vi "test - NESTED Multiple nested read and write operations of submodules.vi"(8 "error in (no error)":errorcluster, 11 "TestCase in":refnum<class "csm-ini-variable-addon.lvclass">) -> (0 "error out":errorcluster, 3 "TestCase out":refnum<class "csm-ini-variable-addon.lvclass">)   [LabVIEW 2017, in "csm-ini-variable-addon.lvclass"]
uses:
  csm-ini-variable-addon.lvclass
  fd1f1403-f650-4147-a5d0-7fa8994ff20a.vi
  a890fef7-7f1d-42c9-b9db-12bb2b441289.vi
  25df91f5-a8e9-4b30-a15a-ad417606420d.vi
  4506128f-911b-4b09-9ad5-a28d51cf287f.vi
  fd1f1403-f650-4147-a5d0-7fa8994ff20a.vi/caddadbc-c5ad-445f-bfd7-34f99667ea02.vi
  <vilib>/Utility/error.llb/Clear Errors.vi
  a890fef7-7f1d-42c9-b9db-12bb2b441289.vi/5b17a956-d3a2-4fc5-bd5f-1f511fac3c4f.vi
  25df91f5-a8e9-4b30-a15a-ad417606420d.vi/a3ec2e19-b962-4b46-9572-7cb078ba8762.vi
  4506128f-911b-4b09-9ad5-a28d51cf287f.vi/14c6159a-6b3d-4974-8c79-afba77de3931.vi
  <vilib>/Utility/Data Type/Get Type Information.vi
  <userlib>/_NEVSTOP/Communicable State Machine(CSM)/addons/API-String-Arugments-Support/_Support/Data To SingleElementsArray_csm.vi
  <userlib>/_NEVSTOP/Communicable State Machine(CSM)/addons/API-String-Arugments-Support/_Support/Data To API String Arguments.vi
  INI-Static-Variable-Support/_Support/Parse Used Session and Name.vi
  INI-Static-Variable-Support/_Support/INI-FGV.vi
  INI-Static-Variable-Support/INI-Static-Variable-Support.lvlib
panel:
  out "text":string
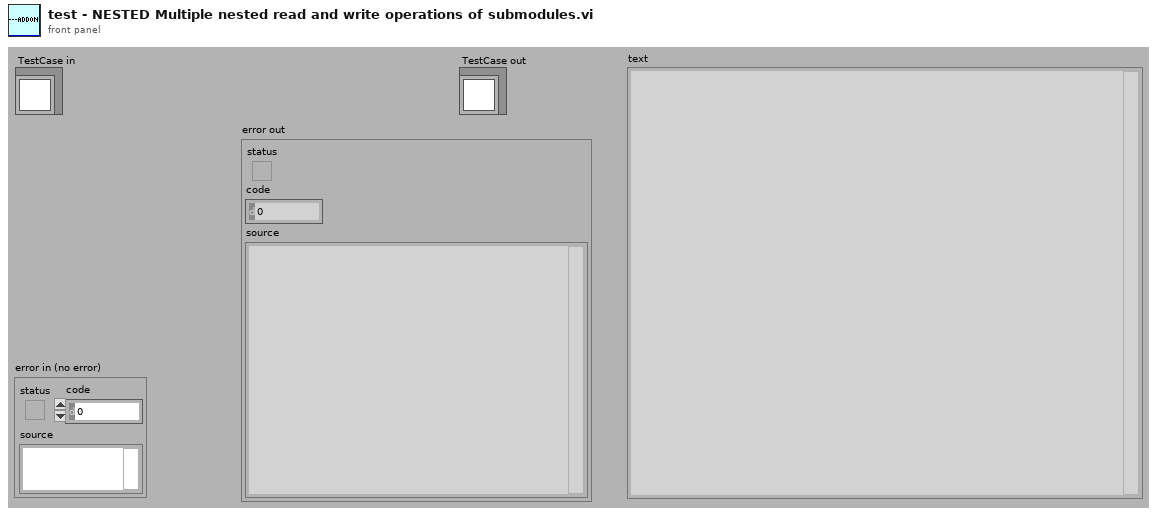
[diagram p1: front panel]
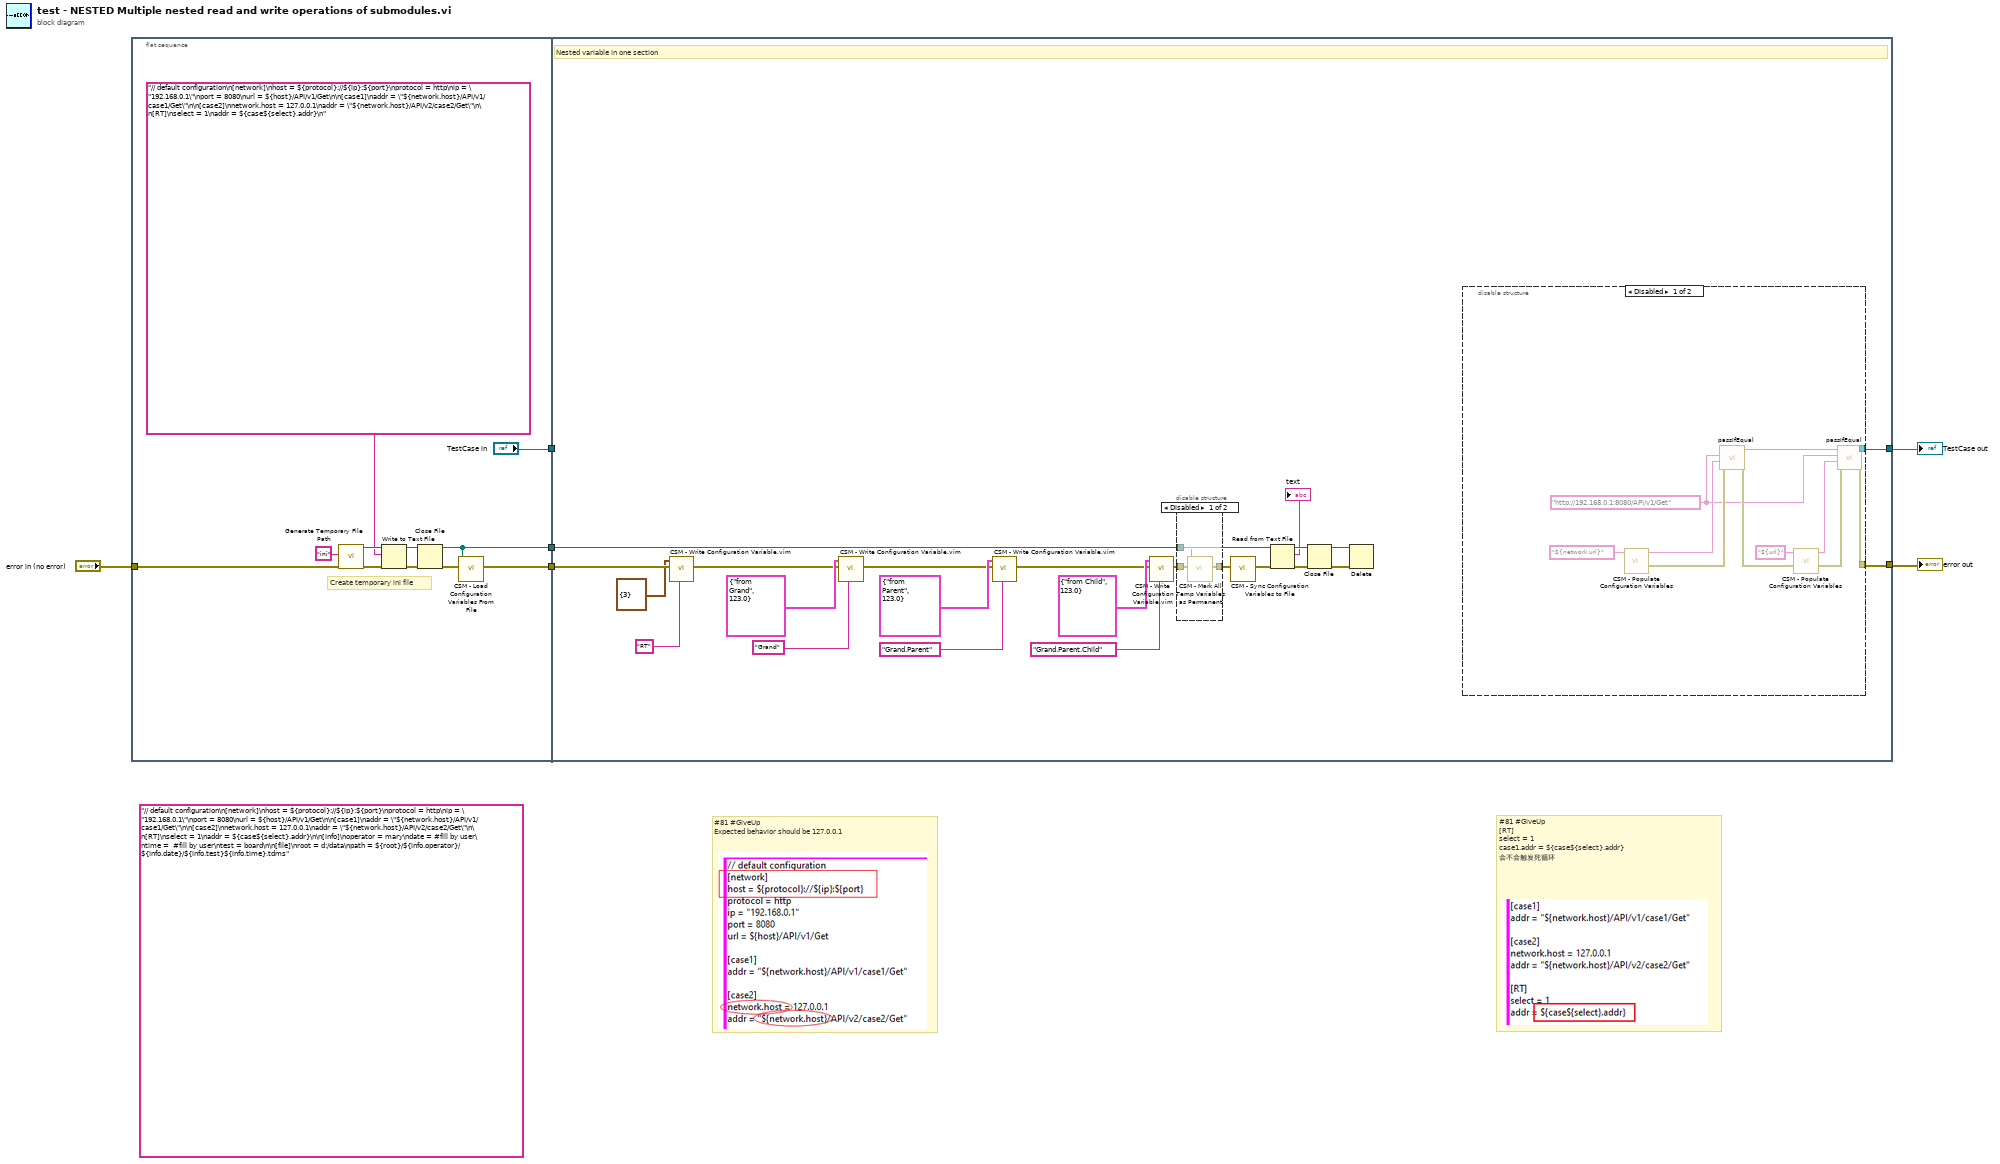
[diagram p0: block diagram]
diagram:
  (unwired) "// default configuration\n[network]\nhost = ${protocol}://${ip}:${port}\nprotocol = http\nip = \"192.168.0.1\"\nport = 8080\nurl = ${host}/API/v1/Get\n\n[case1]\naddr = \"${network.host}/API/v1/case1/Get\"\n\n[case2]\nnetwork.host = 127.0.0.1\naddr = \"${network.host}/API/v2/case2/Get\"\n\n[RT]\nselect = 1\naddr = ${case${select}.addr}\n\n[info]\noperator = mary\ndate = #fill by user\ntime =  #fill by user\ntest = board\n\n[file]\nroot = d:/data\npath = ${root}/${info.operator}/${info.date}/${info.test}${info.time}.tdms"
  # "#81 #GiveUp\nExpected behavior should be 127.0.0.1"
  # "#81 #GiveUp\n[RT]\nselect = 1\ncase1.addr = ${case${select}.addr}\n会不会触发死循环"
  n1 = flat-sequence {
    tunnel: "error in (no error)" -> [w10]
    tunnel: [w8] -> w5
    tunnel: ["TestCase in"] -> w4
    tunnel: [w7] -> w1
    tunnel: w5 -> [w20]
    tunnel: w4 -> [_]
    tunnel: [w40] -> w3
    tunnel: [w39] -> w2
    tunnel: w1 -> [w27]
    frame #0 {
      # "Create temporary ini file"
      n2 = call <vilib>:"Generate Temporary File Path.vi"("error in (no error)"=w10, "Temporary File Extension (tmp)"="ini") -> ("error out"=w17:errorcluster, "Unique Temporary File Path"=w14:path)  [unwired: 8 in]
      n3 = Write to Text File(file (use dialog)=w14, text="// default configuration\n[network]\nhost = ${protocol}://${ip}:${port}\nprotocol = http\nip = \"192.168.0.1\"\nport = 8080\nurl = ${host}/API/v1/Get\n\n[case1]\naddr = \"${network.host}/API/v1/case1/Get\"\n\n[case2]\nnetwork.host = 127.0.0.1\naddr = \"${network.host}/API/v2/case2/Get\"\n\n[RT]\nselect = 1\naddr = ${case${select}.addr}\n", error in=w17) -> (refnum out=w13:refnum<file>, error out=w15:errorcluster)  [unwired: 1 in, 1 out]
      n4 = Close File(refnum=w13, error in=w15) -> (path=w7:path, error out=w12:errorcluster)
      n5 = call "CSM - Load Configuration Variables From File.vi"("error in (no error)"=w12, "Path"=w7) -> ("error out"=w8:errorcluster)  [unwired: 7 in]
    }
    frame #1 {
      # "Nested variable in one section"
      n6 = call "CSM - Write Configuration Variable.vim"("Section Name(\"\" as Default)"="RT" ("Section Name(\"\" as Default)"), "error in (no error)"=w20, "Variant"=cluster{"select":i32} {"select"=3}) -> ("error out"=w21:errorcluster)  [unwired: 5 in, 1 out]
      n7 = call "CSM - Write Configuration Variable.vim"("Section Name(\"\" as Default)"="Grand" ("Section Name(\"\" as Default)"), "error in (no error)"=w21, "Variant"=cluster{"ParamString":string, "ParamDBL":dbl} {"ParamString"="from Grand", "ParamDBL"=123.0}) -> ("error out"=w34:errorcluster)  [unwired: 5 in, 1 out]
      n8 = call "CSM - Write Configuration Variable.vim"("Section Name(\"\" as Default)"="Grand.Parent" ("Section Name(\"\" as Default)"), "error in (no error)"=w34, "Variant"=cluster{"ParamString":string, "ParamDBL":dbl} {"ParamString"="from Parent", "ParamDBL"=123.0}) -> ("error out"=w31:errorcluster)  [unwired: 5 in, 1 out]
      n9 = call "CSM - Write Configuration Variable.vim"("Section Name(\"\" as Default)"="Grand.Parent.Child" ("Section Name(\"\" as Default)"), "error in (no error)"=w31, "Variant"=cluster{"ParamString":string, "ParamDBL":dbl} {"ParamString"="from Child", "ParamDBL"=123.0}) -> ("error out"=w30:errorcluster)  [unwired: 5 in, 1 out]
      n10 = disable-structure shown="Disabled" {
        disable-tunnel: w30 -> [w43 w44]
        disable-tunnel: [w42 w44] -> w29
        disable-tunnel: w27 -> [w41 _]
        frame Disabled {
          n11 = call "CSM - Mark All Temp Variables as Permanent.vi"("error in (no error)"=w43, "Path(\"\" to use default ini)"=w41) -> ("error out"=w42:errorcluster)  [unwired: 7 in]
        }
        frame Enabled {
        }
      }
      n12 = call "CSM - Sync Configuration Variables to File.vi"("error in (no error)"=w29) -> ("error out"=w28:errorcluster)  [unwired: 8 in]
      n13 = Read from Text File(file (use dialog)=w27, error in=w28) -> (refnum out=w26:refnum<file>, text=→"text":string, error out=w25:errorcluster)  [unwired: 2 in, 1 out]
      n14 = Close File(refnum=w26, error in=w25) -> (path=w23:path, error out=w24:errorcluster)
      n15 = Delete(path (use dialog)=w23, error in=w24) -> ()  [unwired: 3 in, 3 out]
      n16 = disable-structure shown="Disabled" {
        disable-tunnel: [w47 _] -> w40
        disable-tunnel: [w46 _] -> w39
        frame Disabled {
          w49 = "http://192.168.0.1:8080/API/v1/Get" ("${network.url}")
          n17 = call "CSM - Populate Configuration Variables.vi"("String in"="${network.url}") -> ("error out"=w53:errorcluster, "String out"=w54:string, "error in (no error)"=w56:errorcluster)  [unwired: 6 in]
          n18 = call-dynamic "passIfEqual.vi"("error in (no error)"=w53, "y"=w54, "x"=w49) -> ("error out"=w52:errorcluster, "TestCase out"=w51:refnum<class "csm-ini-variable-addon.lvclass">, "TestCase in"=w55:refnum<class "csm-ini-variable-addon.lvclass">)  [unwired: 6 in]
          n19 = call "CSM - Populate Configuration Variables.vi"("error in (no error)"=w52, "String in"="${url}") -> ("error out"=w50:errorcluster, "String out"=w48:string, "Section Name(\"\" as Default)"=w45:string)  [unwired: 5 in]
          n20 = call-dynamic "passIfEqual.vi"("error in (no error)"=w50, "y"=w48, "x"=w49, "TestCase in"=w51) -> ("error out"=w46:errorcluster, "TestCase out"=w47:refnum<class "csm-ini-variable-addon.lvclass">)  [unwired: 6 in]
        }
        frame Enabled {
        }
      }
    }
  }
  "error out" <- w2
  "TestCase out" <- w3
